vi "MissionLocation.vi"(8 "Error In":errorcluster, 11 "RoundBouy in":refnum<class "RoundBouy.lvclass">) -> (0 "Error Out":errorcluster, 2 "element":T1 {"North" format="%#_10f"; "East" format="%#_8f"}, 3 "RoundBouy out":refnum<class "RoundBouy.lvclass">)   [LabVIEW 2013, in "RoundBouy.lvclass"]
uses:
  RoundBouy.lvclass
  Data/TypeDefs/UTM Location.ctl
  GenericMission/GenericMission.lvclass
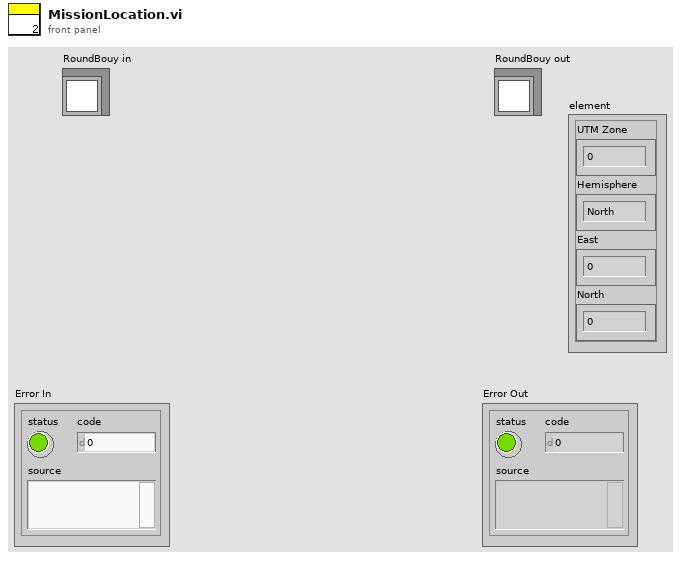
[diagram p1: front panel]
types:
  T1 = typedef "UTM Location.ctl" = cluster{"UTM Zone":dbl, "Hemisphere":enum16{"North", "South"}, "East":dbl, "North":dbl}
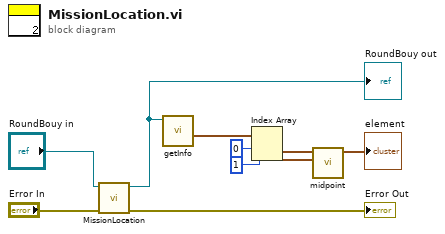
[diagram p0: block diagram]
diagram:
  n1 = call-parent "MissionLocation.vi"("Error In"="Error In", "GenericMission in"="RoundBouy in") -> ("Error Out"=→"Error Out":errorcluster, "GenericMission out"=w2:refnum<class "RoundBouy.lvclass">)  [unwired: 7 in, 1 out]
  "RoundBouy out" <- w2
  n2 = call-dynamic "getInfo.vi"("GenericMission in"=w2) -> ("Points of Interest"=w3:T1[])  [unwired: 3 in, 7 out]
  n3 = Index Array(array=w3, index #1=0 ("index"), index #2=1 ("index")) -> (element #1=w5:T1, element #2=w4:T1)
  n4 = call "midpoint.vi"("UTM Location 2"=w4, "UTM Location"=w5) -> ("UTM Location 3"=→"element":T1)  [unwired: 8 in, 1 out]
